vi "Salva_Calagem_Global.vi"   [LabVIEW 2018]
uses:
  Global_Telescopio.vi
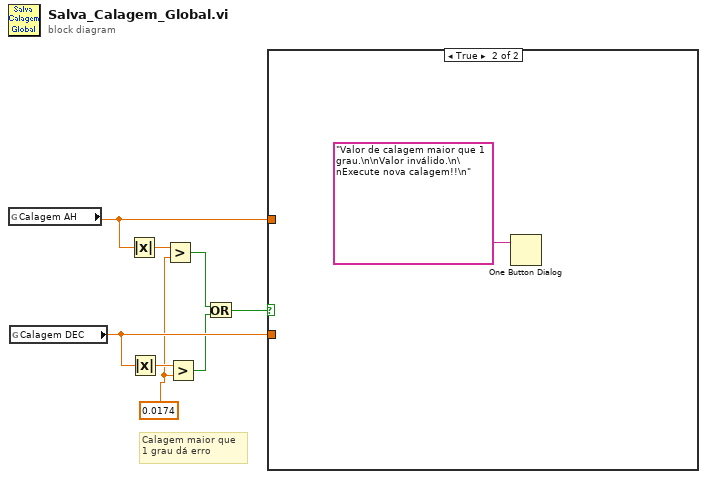
[diagram p0: block diagram]
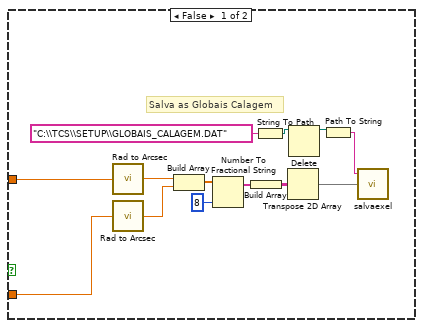
[diagram p2: hidden frame]
diagram:
  w1 = 0.0174 ("Calagem DEC")
  # "Calagem maior que\n1 grau dá erro"
  n1 = global read "Global_Telescopio.vi" "Calagem AH"() -> (w7:dbl)
  n2 = global read "Global_Telescopio.vi" "Calagem DEC"() -> (w8:dbl)
  n3 = Absolute Value(x=w7) -> (abs(x)=w6:dbl)
  n4 = Absolute Value(x=w8) -> (abs(x)=w5:dbl)
  n5 = Greater?(x=w6, y=w1) -> (0:w4:bool)
  n6 = Greater?(x=w5, y=w1) -> (0:w3:bool)
  n7 = Or(x=w4, y=w3) -> (x .or. y?=w2:bool)
  n8 = case shown="True" w2 {
    tunnel: w8 -> [w10 _]
    tunnel: w7 -> [w9 _]
    frame False {
      # "Salva as Globais Calagem"
      n9 = call "Rad to Arcsec.vi"("Radiano"=w9) -> ("Arcsec"=w11:dbl)
      n10 = call "Rad to Arcsec.vi"("Radiano"=w10) -> ("Arcsec"=w12:dbl)
      n11 = Build Array(w11, w12) -> (w19:dbl[])
      n12 = Number To Fractional String(number=w19, precision (6)=i16 8) -> (F-format string=w20:string[])  [unwired: 2 in]
      n13 = Build Array(w20) -> (w14:string[][])
      n14 = String To Path(string="C:\\TCS\\SETUP\\GLOBAIS_CALAGEM.DAT") -> (path=w15:path)
      n15 = Transpose 2D Array(2D array=w14) -> (transposed array=w13:string[][])
      n16 = Delete(path (use dialog)=w15) -> (deleted path=w16:path)  [unwired: 4 in, 2 out]
      n17 = Path To String(path=w16) -> (string=w17:string)
      n18 = call "salvaexel.vi"("appended array"=w13, "file name p/ exell"=w17) -> ()  [unwired: 1 in, 1 out]
    }
    frame True {
      n19 = One Button Dialog(message="Valor de calagem maior que 1 grau.\n\nValor inválido.\n\nExecute nova calagem!!\n") -> ()  [unwired: 1 in, 1 out]
    }
  }
